vi "daqio_Write_Multiple_single_Timestamp.vi"(7 "daq.io Device Channel Keys":string[](array[string]), 8 "error in (no error)":errorcluster, 9 "Timestamp":timestamp, 10 "Values":dbl[](array[numeric]), 11 "daq.io type in":T1={"daq.io ref"=refnum, "daq.io API Base"="http://dashboard.daq.io/api/v1", "Device Type Key"="", "Device Key"="", "Account ID"="", "online"=FALSE}) -> (0 "error out":errorcluster, 3 "daq.io type out":T1={"daq.io ref"=refnum, "daq.io API Base"="http://dashboard.daq.io/api/v1", "Device Type Key"="", "Device Key"="", "Account ID"="", "online"=FALSE})   [LabVIEW 2013, in "daqio minimal.lvlib"]
doc: "This VI writes multiple data points to a channel of a daq.io device with the same time stamp. \n\nIf the daq.io Device Channel does not exist online, a new channel will be auto-created and data will be stored there. You have to provide a Channel Key where the value will be written to."
uses:
  daqio minimal.lvlib
  _typedefs/daqio-Type.ctl
  <vilib>/httpClient/ClientHandle.ctl
  _typedefs/FGV_commands.ctl
  _typedefs/daqio-TimeSeriesEntry.ctl
  _typedefs/daqio-Buffer-Commands.ctl
  _typedefs/connection_FGV_commands.ctl
  <vilib>/Easy HTTP Client/Easy HTTP.lvlib
  <vilib>/httpClient/LabVIEWHTTPClient.lvlib
panel:
  out "JSON string":string
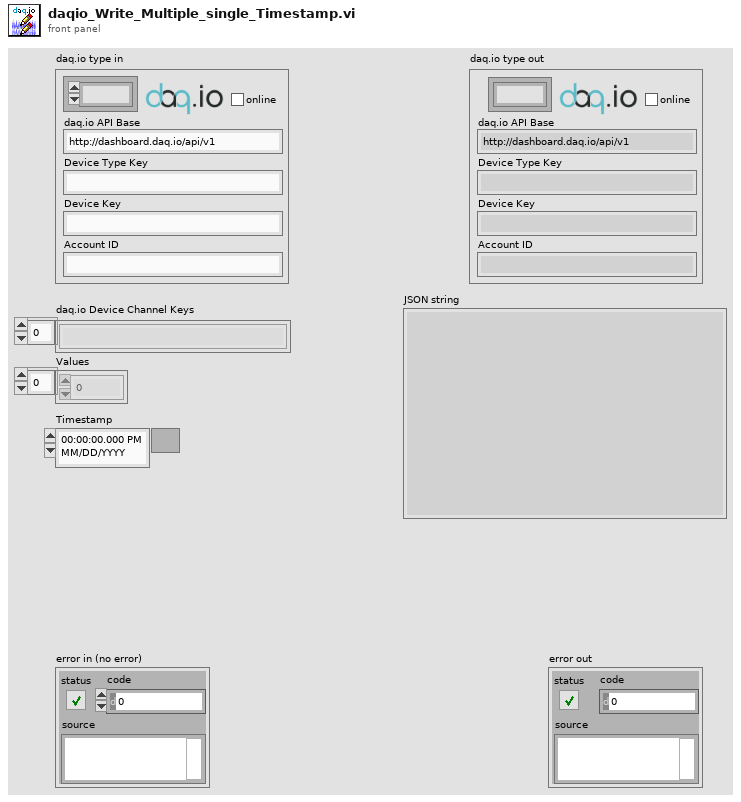
[diagram p1: front panel]
types:
  T1 = typedef "daqio minimal.lvlib/daqio-Type.ctl" = cluster{"daq.io ref":T2, "daq.io API Base":string, "Device Type Key":string, "Device Key":string, "Account ID":string, "online":bool}
  T2 = typedef "LabVIEWHTTPClient.lvlib/ClientHandle.ctl" = refnum<k1>
  T3 = typedef "daqio minimal.lvlib/daqio-TimeSeriesEntry.ctl" = cluster{"channel_type_id":string, "device_id":string, "time":string, "value":dbl}
  T4 = typedef "daqio minimal.lvlib/FGV_commands.ctl" = enum16{"Init / update", "Edit Item", "Find or Add Item", "Remove Item", "Delete All"}
  T5 = typedef "daqio minimal.lvlib/daqio-Buffer-Commands.ctl" = enum16{"Add to Buffer", "Post from Buffer", "Clear Buffer", "Init"}
  T6 = typedef "daqio minimal.lvlib/connection_FGV_commands.ctl" = enum16{"Set Conn Stat", "Set Type", "Set Buffer", "Get"}
  T7 = typedef "daqio minimal.lvlib/daqio-Device-Type-Info-return.ctl" = cluster{"channel_types":T8[], "devices":T9[], "label":string, "event_types":T10[], "key":string, "tag_types":T11[], "id":string, "permissions":cluster{"write":string[], "read":string[]}}
  T8 = typedef "daqio minimal.lvlib/daqio-Channel-Type-POST-return.ctl" = cluster{"device_type_id":string, "id":string, "key":string, "label":string, "data_type":string, "permissions":cluster{"write":string[], "read":string[]}}
  T9 = typedef "daqio minimal.lvlib/daqio-Device.ctl" = cluster{"permissions":cluster{"write":string[], "read":string[]}, "id":string, "label":string, "key":string, "device_type_id":string, "tags":cluster{"key":string, "value":string}[], "files":string[]}
  T10 = typedef "daqio minimal.lvlib/daqio-Event-Type.ctl" = cluster{"device_type_id":string, "permissions":cluster{"read":string[], "write":string[]}, "id":string, "key":string, "label":string}
  T11 = typedef "daqio minimal.lvlib/daqio-Tag-Type-POST-return.ctl" = cluster{"label":string, "id":string, "device_type_id":string, "permissions":cluster{"write":string[], "read":string[]}, "default":string, "key":string}
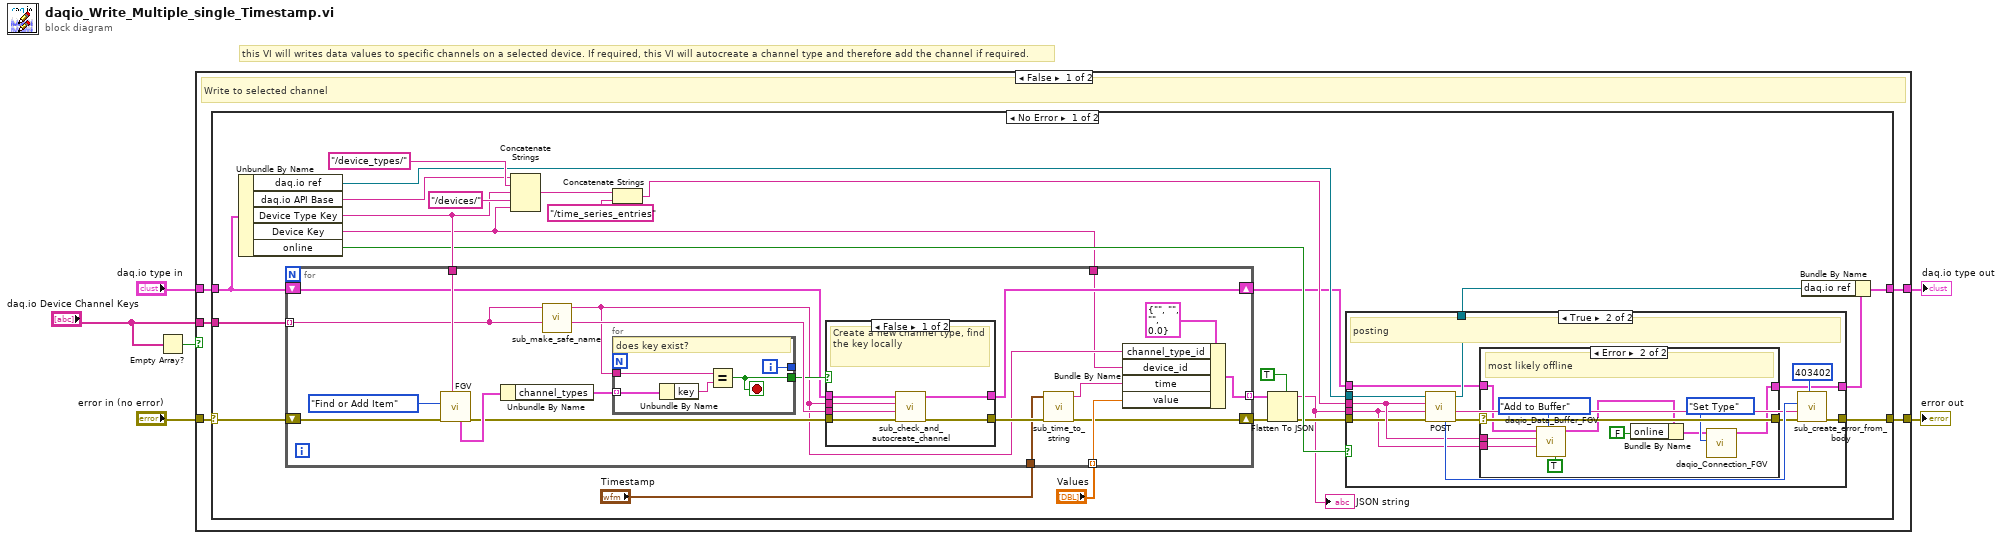
[diagram p0: block diagram]
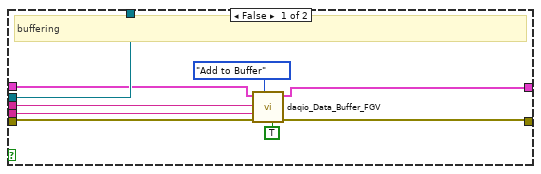
[diagram p3: hidden frame]
diagram:
  # "this VI will writes data values to specific channels on a selected device. If required, this VI will autocreate a channel type and therefore add the channel if required."
  n1 = Empty Array?(array="daq.io Device Channel Keys") -> (empty?=w3:bool)
  n2 = case shown="False" w3 {
    tunnel: "daq.io type in" -> [w11 w107]
    tunnel: [w10 w107] -> w6
    tunnel: [w9 w106] -> w5
    tunnel: "error in (no error)" -> [w8 w106]
    tunnel: "daq.io Device Channel Keys" -> [w7 _]
    frame False {
      # "Write to selected channel"
      n3 = case shown="No Error" w8 {
        selector: w8 -> [w25 w104]
        tunnel: w11 -> [w15 w105]
        tunnel: [w14 w105] -> w10
        tunnel: [w26 w104] -> w9
        tunnel: w7 -> [w27 _]
        frame No Error {
          n4 = Unbundle By Name(w15) -> ("daq.io ref"=w29:T2, "daq.io API Base"=w34:string, "Device Type Key"=w28:string, "Device Key"=w21:string, "online"=w24:bool)
          n5 = for {
            tunnel: w28 -> [w52]
            tunnel: w27 -> [w51] mode=indexing
            shift-right: [w37] -> w19
            shift-left: w25 -> [w48]
            shift-right: [w44] -> w23
            shift-left: w15 -> [w45]
            tunnel: "Timestamp" -> [w43]
            tunnel: "Values" -> [w42] mode=indexing
            tunnel: w21 -> [w41]
            tunnel: [w38] -> w20 mode=indexing
            n6 = call "FGV.vi"("Dev Type Key"=w52, "error in (no error)"=w48, "Action"=FGV_commands."Find or Add Item") -> ("error out"=w47:errorcluster, "Dev Type out"=w54:T7)  [unwired: 4 in, 3 out]
            n7 = Unbundle By Name(w54) -> ("channel_types"=w55:T8[])
            n8 = call "sub_make_safe_name.vi"("Input String"=w51) -> ("Safe Output String"=w46:string)  [unwired: 10 in]
            n9 = for {
              tunnel: w55 -> [w68] mode=indexing
              tunnel: w46 -> [w65]
              tunnel: [w67] -> w49
              tunnel: [w66] -> _
              i -> [w66]
              stop <- w67 stop-if-true
              # "does key exist?"
              n10 = Unbundle By Name(w68) -> ("key"=w64:string)
              n11 = Equal?(x=w65, y=w64) -> (x = y?=w67:bool)
            }
            n12 = case shown="False" w49 {
              tunnel: [w61 w63] -> w44
              tunnel: [w56 w62] -> w50
              tunnel: w46 -> [w59 _]
              tunnel: w45 -> [w60 w63]
              tunnel: w51 -> [w58 _]
              tunnel: w47 -> [w57 w62]
              frame False {
                # "Create a new channel type, find the key locally"
                n13 = call "sub_check_and_autocreate_channel.vi"("error in (no error)"=w57, "daq.io Device Channel Label"=w58, "daq.io Device Channel Key to write to"=w59, "daq.io type in in"=w60) -> ("error out"=w56:errorcluster, "daq.io type out"=w61:T1)  [unwired: 5 in, 1 out]
              }
              frame True {
                # "Key was found in the existing device types"
              }
            }
            n14 = call "sub_time_to_string.vi"("error in (no error)"=w50, "timestamp"=w43) -> ("error out"=w37:errorcluster, "time"=w40:string)  [unwired: 8 in]
            n15 = Bundle By Name(cluster=T3 {"channel_type_id"="", "device_id"="", "time"="", "value"=0.0}, "channel_type_id"=w46, "device_id"=w41, "time"=w40, "value"=w42) -> (w38:T3)
          }
          n16 = Concatenate Strings(w34, "/device_types/", w28, "/devices/", w21) -> (w30:string)
          n17 = Concatenate Strings(w30, "/time_series_entries") -> (w31:string)
          n18 = Flatten To JSON(enable LabVIEW extensions? (T)=TRUE, anything=w20, error in (no error)=w19) -> (JSON string=w16:string, 11:w17:errorcluster)
          "JSON string" <- w16
          n19 = case shown="True" w24 {
            tunnel: [w77 w90] -> w33
            tunnel: w31 -> [w75 w81]
            tunnel: w29 -> [w77 w89]
            tunnel: [w76 w88] -> w26
            tunnel: w23 -> [w73 w83]
            tunnel: [w71 w82] -> w13
            tunnel: w17 -> [w70 w79]
            tunnel: w16 -> [w72 w78]
            frame False {
              # "buffering"
              n20 = call "daqio_Data_Buffer_FGV.vi"("Is Array?"=TRUE, "Buffer Command"=daqio-Buffer-Commands."Add to Buffer", "error in (no error)"=w70, "JSON Data"=w72, "API route"=w75, "daq.io type in"=w73) -> ("error out"=w76:errorcluster, "daq.io type out"=w71:T1)  [unwired: 4 in]
            }
            frame True {
              # "posting"
              n21 = call <vilib>:"POST.vi"("error in (no error)"=w79, "data"=w78, "url"=w81, "client handle"=w89) -> ("error out"=w84:errorcluster, "body"=w85:string, "client handle out"=w90:T2, "HTTP Response Code"=w87:i32)  [unwired: 3 in, 1 out]
              n22 = case shown="Error" w84 {
                selector: w84 -> [w92 w103]
                tunnel: [w92 w103] -> w80
                tunnel: [w91 w93] -> w82
                tunnel: w83 -> [w91 w94]
                tunnel: w81 -> [_ w97]
                tunnel: w78 -> [_ w96]
                frame No Error {
                }
                frame Error {
                  # "most likely offline"
                  n23 = call "daqio_Data_Buffer_FGV.vi"("Is Array?"=TRUE, "Buffer Command"=daqio-Buffer-Commands."Add to Buffer", "JSON Data"=w96, "API route"=w97, "daq.io type in"=w94) -> ("daq.io type out"=w100:T1)  [unwired: 5 in, 1 out]
                  n24 = Bundle By Name(cluster=w100, "online"=FALSE) -> (w98:T1)
                  n25 = call "daqio_Connection_FGV.vi"("Enum"=connection_FGV_commands."Set Type", "daq.io type in"=w98) -> ("daq.io type out"=w93:T1)  [unwired: 6 in, 3 out]
                }
              }
              n26 = call "sub_create_error_from_body.vi"("error code"=403402, "error in (no error)"=w80, "http code"=w87, "body"=w85) -> ("error out"=w88:errorcluster)  [unwired: 7 in]
            }
          }
          n27 = Bundle By Name(cluster=w13, "daq.io ref"=w33) -> (w14:T1)
        }
        frame Error {
        }
      }
    }
    frame True {
      # "no Channel Key: nothing to do"
    }
  }
  "error out" <- w5
  "daq.io type out" <- w6
